vi "Add Entry DBL.vi"(6 "Result":T1, 8 "error in (no error)":errorcluster, 9 "Value DBL":dbl, 10 "Name":string, 11 "Results in":refnum<class "Results.lvclass">) -> (0 "error out":errorcluster, 3 "Results out":refnum<class "Results.lvclass">)   [LabVIEW 2020, in "Tester.lvlib" / "Results.lvclass"]
uses:
  Results.lvclass
  Result.ctl
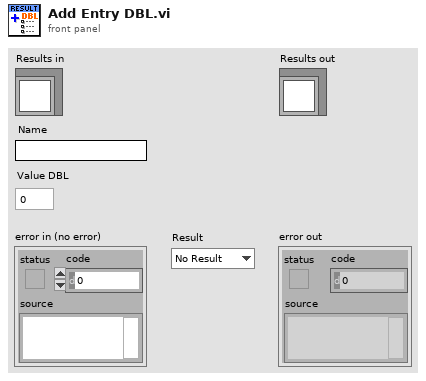
[diagram p1: front panel]
types:
  T1 = typedef "Tester.lvlib/Results.lvclass/Result.ctl" = enum16{"No Result", "Pass", "Fail", "Error", "Abort"}
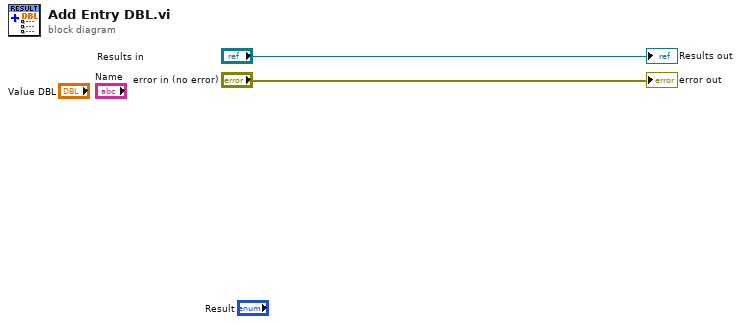
[diagram p0: block diagram]
diagram:
  "error out" <- "error in (no error)"
  "Results out" <- "Results in"
